vi "UDP Vision - Receiver.vi"(11 "receiver port":u16=1180) -> (3 "Image":T1(plugin-control))   [LabVIEW 2019]
doc: "The UDP protocol differs from TCP in that there is no error-checking with the packets of information that are sent, and thus no guarantee whatsoever that an intended recipient will actually receive a given piece of data.\n\nUDP does offer the ability to \"broadcast\" data across a network--simply specify an IP Address of all ones (255.255.255.255) to attempt to broadcast information network-wide. Keep in mind that routers and other network hardware will generally refuse to forward the broadcast beyond certain points, so the extent of the broadcast will in practice be limited."
uses:
  <vilib>/vision/Image Controls.llb/IMAQ Image.ctl
panel:
  in  "Stop":bool
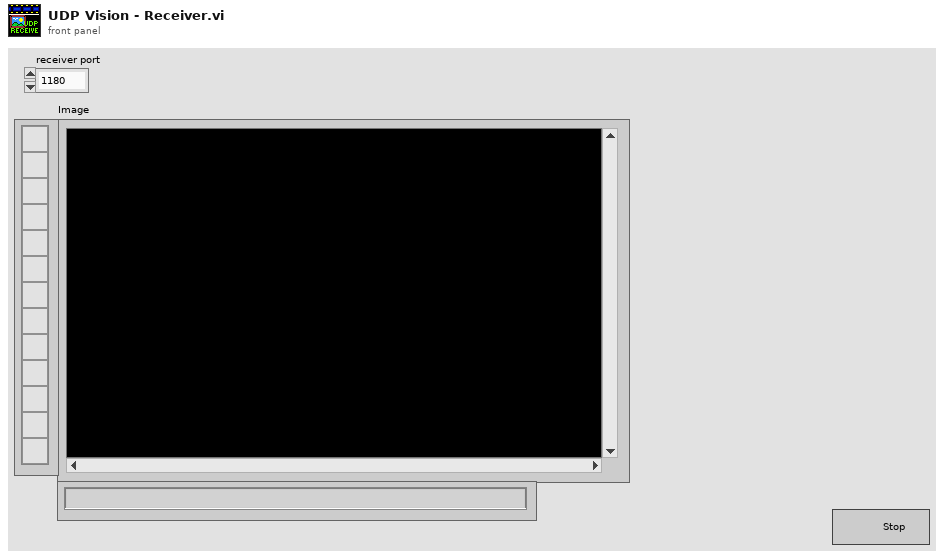
[diagram p1: front panel]
types:
  T1 = typedef "IMAQ Image.ctl" = refnum<image>
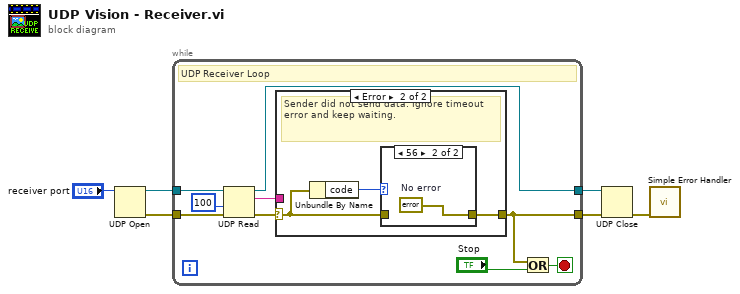
[diagram p0: block diagram]
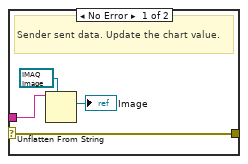
[diagram p2: hidden frame]
diagram:
  n1 = UDP Open(11:"receiver port") -> (port=w2:refnum<k16>, 0:w3:errorcluster)  [unwired: 4 in, 1 out]
  n2 = while {
    tunnel: w2 -> [w15]
    tunnel: [w7] -> w6
    tunnel: w3 -> [w12]
    tunnel: [w8] -> w4
    stop <- w13 stop-if-true
    # "UDP Receiver Loop"
    n3 = UDP Read(connection ID=w15, timeout ms (25000)=100, 8:w12) -> (data out=w10:string, error out=w9:errorcluster, 3:w7:refnum<k16>)  [unwired: 3 out]
    n4 = case shown="Error" w9 {
      selector: w9 -> [w19 w21]
      tunnel: w10 -> [w18 _]
      tunnel: [w19 w20] -> w8
      frame No Error {
        # "Sender sent data. Update the chart value."
        n5 = Unflatten From String(type=T1 refnum ("Image Out"), binary string=w18) -> (value=→"Image":T1)  [unwired: 3 in, 2 out]
      }
      frame Error {
        # "Sender did not send data. Ignore timeout error and keep waiting."
        n6 = Unbundle By Name(w21) -> ("code"=w22:i32)
        n7 = case shown="56" w22 {
          tunnel: w21 -> [w23 _]
          tunnel: [w23 w24] -> w20
          frame Default {
          }
          frame 56 {
            w24 = errorcluster {"status"=FALSE, "code"=0, "source"=""}  # No error
          }
        }
      }
    }
    n8 = Or(x=w8, y="Stop") -> (x .or. y?=w13:bool)
  }
  n9 = UDP Close(connection ID=w6, 8:w4) -> (error out=w5:errorcluster)  [unwired: 1 out]
  n10 = call <vilib>:"Simple Error Handler.vi"("error in (no error)"=w5) -> ()  [unwired: 1 in, 8 out]
